vi "Add Variant to JSON Object.vi"(7 "Treatment of Infinity/NaN":T1, 8 "error in (no error)":errorcluster, 10 "Variant":variant, 11 "JSON Object in":refnum<class "JSON Object.lvclass">) -> (0 "error out":errorcluster, 3 "JSON Object out":refnum<class "JSON Object.lvclass">)   [LabVIEW 2011, in "Variant JSON.lvlib"]
doc: "Adds a Variant to a JSON object. Variant data name will be used as the item name (unnamed data is ignored). Clusters are converted to JSON objects. Variants, if empty (void), are converted to null, unless they have attributes, in which case these are converted into a JSON object. \n\nTreatment of Infinity, -Infinity, and Not-a-Number values of floating-point numerics:\n<b>-- Default JSON:</b> write all as nulls.\n<b>-- Extended:</b> use JSON strings for Infinities (\"Infinity\", \"-Infinity\"); NaN still null.\n<b>-- LabVIEW extentions</b> (compatable with the LabVIEW JSON primatives): Infinity, -Infinity, NaN (not in quotes)"
uses:
  Variant JSON.lvlib
  JSON Scalar/Infinity&NaN.ctl
  JSON Object/JSON Object.lvclass
  <vilib>/Utility/VariantDataType/VariantType.lvlib
  JSON Scalar/JSON Scalar.lvclass
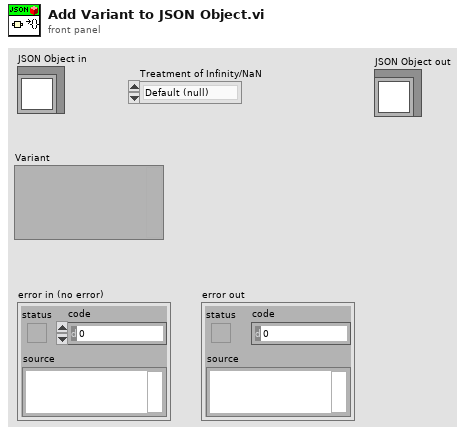
[diagram p1: front panel]
types:
  T1 = typedef "JSON Scalar.lvclass/Infinity&NaN.ctl" = enum16{"Default (null)", "Extended", "LabVIEW extensions"}
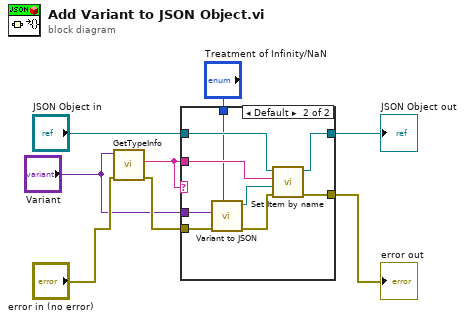
[diagram p0: block diagram]
diagram:
  n1 = call <vilib>:"GetTypeInfo.vi"("error in (no error)"="error in (no error)", "Variant"="Variant") -> ("error out"=w5:errorcluster, "Name"=w7:string)  [unwired: 5 in, 3 out]
  n2 = case shown="Default" w7 {
    tunnel: "JSON Object in" -> [w10 w19]
    tunnel: [w10 w18] -> w2
    tunnel: w7 -> [_ w17]
    tunnel: "Variant" -> [_ w16]
    tunnel: w5 -> [w9 w14]
    tunnel: [w9 w12] -> w6
    tunnel: "Treatment of Infinity/NaN" -> [_ w11]
    frame "" {
      # "unnamed items ignored"
    }
    frame Default {
      n3 = call "Variant to JSON.vi"("Treatment of Infinity/NaN"=w11, "error in (no error)"=w14, "Variant"=w16) -> ("error out"=w13:errorcluster, "JSON Value out"=w15:refnum<class "JSON Value.lvclass">)  [unwired: 7 in]
      n4 = call-dynamic "Set Item by name.vi"("error in (no error)"=w13, "Value"=w15, "name"=w17, "JSON Object in"=w19) -> ("error out"=w12:errorcluster, "JSON Object out"=w18:refnum<class "JSON Object.lvclass">)  [unwired: 5 in, 1 out]
    }
  }
  "error out" <- w6
  "JSON Object out" <- w2
